vi "Stop and Close SV.vi"(8 "error in (no error)":errorcluster, 11 "SV Data":T1={"Status notifier"=refnum, "Write FIFO ref"=refnum, "Read FIFO ref"=refnum, "Update Rate"=1, "Write Refs by Type"={"DBL Write"=[], "Bool Write"=[], "DBLIndex"=[], "BoolIndex"=[]}, "Read Refs by Type"={"DBL Read"=[], "Bool Read"=[], "DBLIndex"=[], "BoolIndex"=[]}, "WriteSize"=0, "ReadSize"=0}) -> (0 "error out":errorcluster, 3 "SV Data":T1)   [LabVIEW 2016, in "Shared Variable Interface.lvlib"]
uses:
  Shared Variable Interface.lvlib
  DataTypes/Bool.lvlib
  DataTypes/DBL.lvlib
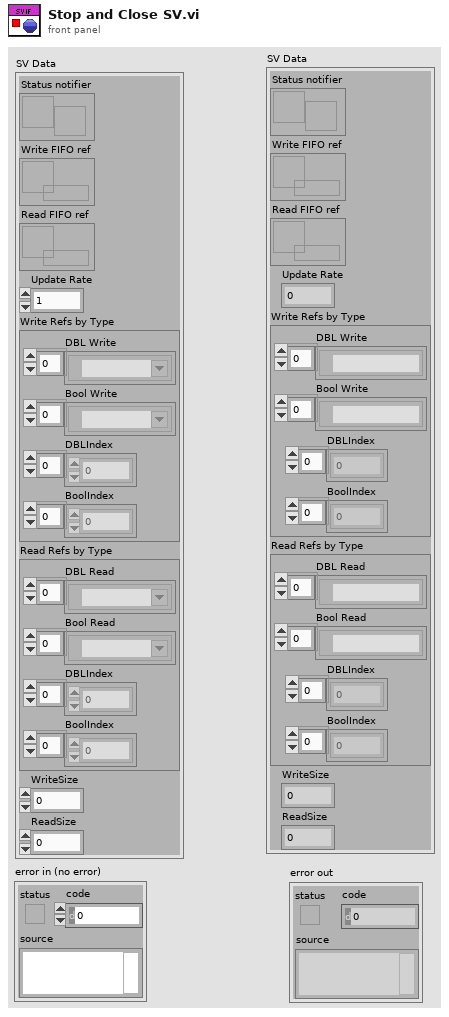
[diagram p1: front panel]
types:
  T1 = cluster{"Status notifier":refnum<notifier>, "Write FIFO ref":refnum<k33>, "Read FIFO ref":refnum<k33>, "Update Rate":u32, "Write Refs by Type":cluster{"DBL Write":refnum<k21>[], "Bool Write":refnum<k21>[], "DBLIndex":i32[], "BoolIndex":i32[]}, "Read Refs by Type":cluster{"DBL Read":refnum<k21>[], "Bool Read":refnum<k21>[], "DBLIndex":i32[], "BoolIndex":i32[]}, "WriteSize":i32, "ReadSize":i32}
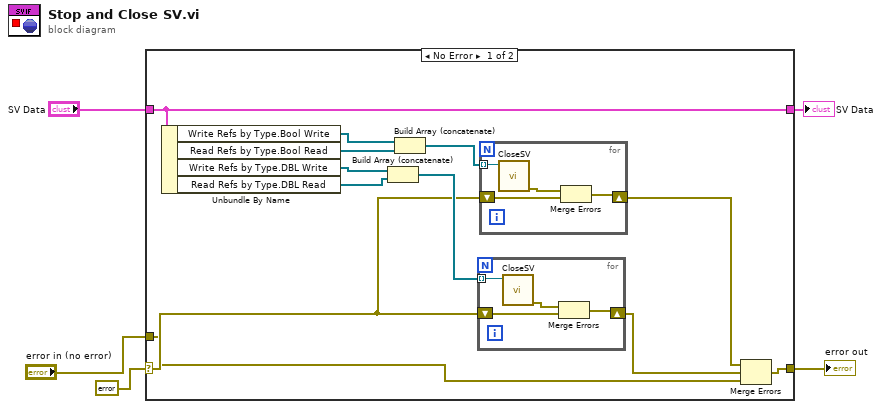
[diagram p0: block diagram]
diagram:
  n1 = case shown="No Error" errorcluster {"status"=FALSE, "code"=0, "source"=""} ("error IO") {
    selector: errorcluster {"status"=FALSE, "code"=0, "source"=""} ("error IO") -> [w12 w27]
    tunnel: [w16 w27] -> w5
    tunnel: "error in (no error)" -> [w11 _]
    tunnel: "SV Data" -> [w6 w26]
    tunnel: [w6 w26] -> w1
    frame No Error {
      n2 = Unbundle By Name(w6) -> ("Write Refs by Type.Bool Write"=w10:refnum<k21>[], "Read Refs by Type.Bool Read"=w9:refnum<k21>[], "Write Refs by Type.DBL Write"=w8:refnum<k21>[], "Read Refs by Type.DBL Read"=w7:refnum<k21>[])
      n3 = Build Array (concatenate)(w8, w7) -> (w14:refnum<k21>[])
      n4 = Build Array (concatenate)(w10, w9) -> (w15:refnum<k21>[])
      n5 = for {
        shift-right: [w20] -> w13
        shift-left: w12 -> [w21]
        tunnel: w14 -> [w18] mode=indexing
        n6 = call "CloseSV.vi"("Shared variable refnum"=w18) -> ("error out"=w19:errorcluster)  [unwired: 10 in]
        n7 = Merge Errors(w19, w21) -> (w20:errorcluster)
      }
      n8 = for {
        tunnel: w15 -> [w22] mode=indexing
        shift-right: [w23] -> w17
        shift-left: w12 -> [w24]
        n9 = call "CloseSV.vi"("shared variable refnum"=w22) -> ("error out"=w25:errorcluster)  [unwired: 10 in]
        n10 = Merge Errors(w25, w24) -> (w23:errorcluster)
      }
      n11 = Merge Errors(w17, w13, w11) -> (w16:errorcluster)
    }
    frame Error {
    }
  }
  "error out" <- w5
  "SV Data" <- w1
